vi "Vigia.vi"(7 "test module":T6, 10 "Robot":T1={"id"=0, "function"=enum."Attacker", "x"=0.0, "y"=0.0, "orientation"=0.0, "v_tangent"=0.0, "v_normal"=0.0, "v_ang"=0.0, "kick_x"=0.0, "kick_z"=0.0, "dribble"=FALSE, "Timestamp"=timestamp(0 s since 1904-01-01), "estimatives"={"est_v_tangent"=0.0, "est_v_normal"=0.0, "est_vx"=0.0, "est_vy"=0.0, "Pos Robot Est"=[]}, "dest_x_kick"=0.0, "dest_y_kick"=0.0, "Gap Coord"=[], "States"=enum."GoToTangent", "Path "=[], "Path  Smooth"=[], "Dest"=[], "Missões "=enum."Monitorar Comboio", "Agentes Disponíveis"=0.0, "Number"=0.0} {"Agentes Disponíveis" format="%#_13g"}, 11 "Al Input":T8={"our_robots"=[], "enemy_robots"=[], "balls"=[], "geometry"={"line_width"=0, "field_length"=0, "field_width"=0, "boundary_width"=0, "referee_width"=0, "goal_width"=0, "goal_depth"=0, "goal_wall_width"=0, "center_circle_radius"=0, "defense_radius"=0, "defense_stretch"=0, "free_kick_from_defense_dist"=0, "penalty_spot_from_field_line_dist"=0, "penalty_line_from_spot_dist"=0}, "IA Judge"={"stage"="", "command"="", "our_goalie_id"=0.0, "enemy_goalie_id"=0.0, "command enum"=enum."Halt", "Time"=enum."Azul"}, "Received Timestamp"=timestamp(0 s since 1904-01-01), "Events"={"Touch"=FALSE, "Ball out"=FALSE, "id touch"=0.0, "Ball out of \nVision"=FALSE, "Ball inside \nGoalie area"=FALSE, "Robot not responding"=FALSE, "Robots responding status"=[1.0, 1.0, 1.0, 1.0, 1.0, 1.0], "Enemy Ball \nPossession"=FALSE, "Pass State"=FALSE, "id end of pass"=0.0, "Kick"=FALSE, "Id ini Possession"=0.0, "Ball Possesion"=FALSE, "Id Possesion"=0.0, "Direct Kick"=FALSE, "2nd Strk Ativo"=FALSE}} {"enemy_robots"."Agentes Disponíveis" format="%#_13g"; "our_robots"."Agentes Disponíveis" format="%#_13g"}) -> (3 "Output Robot":T1={"id"=0, "function"=enum."Attacker", "x"=0.0, "y"=0.0, "orientation"=0.0, "v_tangent"=0.0, "v_normal"=0.0, "v_ang"=0.0, "kick_x"=0.0, "kick_z"=0.0, "dribble"=FALSE, "Timestamp"=timestamp(0 s since 1904-01-01), "estimatives"={"est_v_tangent"=0.0, "est_v_normal"=0.0, "est_vx"=0.0, "est_vy"=0.0, "Pos Robot Est"=[]}, "dest_x_kick"=0.0, "dest_y_kick"=0.0, "Gap Coord"=[], "States"=enum."GoToTangent", "Path "=[], "Path  Smooth"=[], "Dest"=[], "Missões "=enum."Monitorar Comboio", "Agentes Disponíveis"=0.0, "Number"=0.0} {"Agentes Disponíveis" format="%#_13g"})   [LabVIEW 2018]
uses:
  Core/AI Robot.ctl
  Functions Enum.ctl
  AttackerStates.ctl
  Path Planning/RRT/PathDests.ctl
  Path Planning/RRT/PathDest.ctl
  Core/AI Input.ctl
  Core/AI Ball.ctl
  Core/Field Size.ctl
  Core/AI Judge.ctl
  Command Enum.ctl
  Util/Events/Events.ctl
  Test/TestModule.ctl
  Util/Select None or Robot.ctl
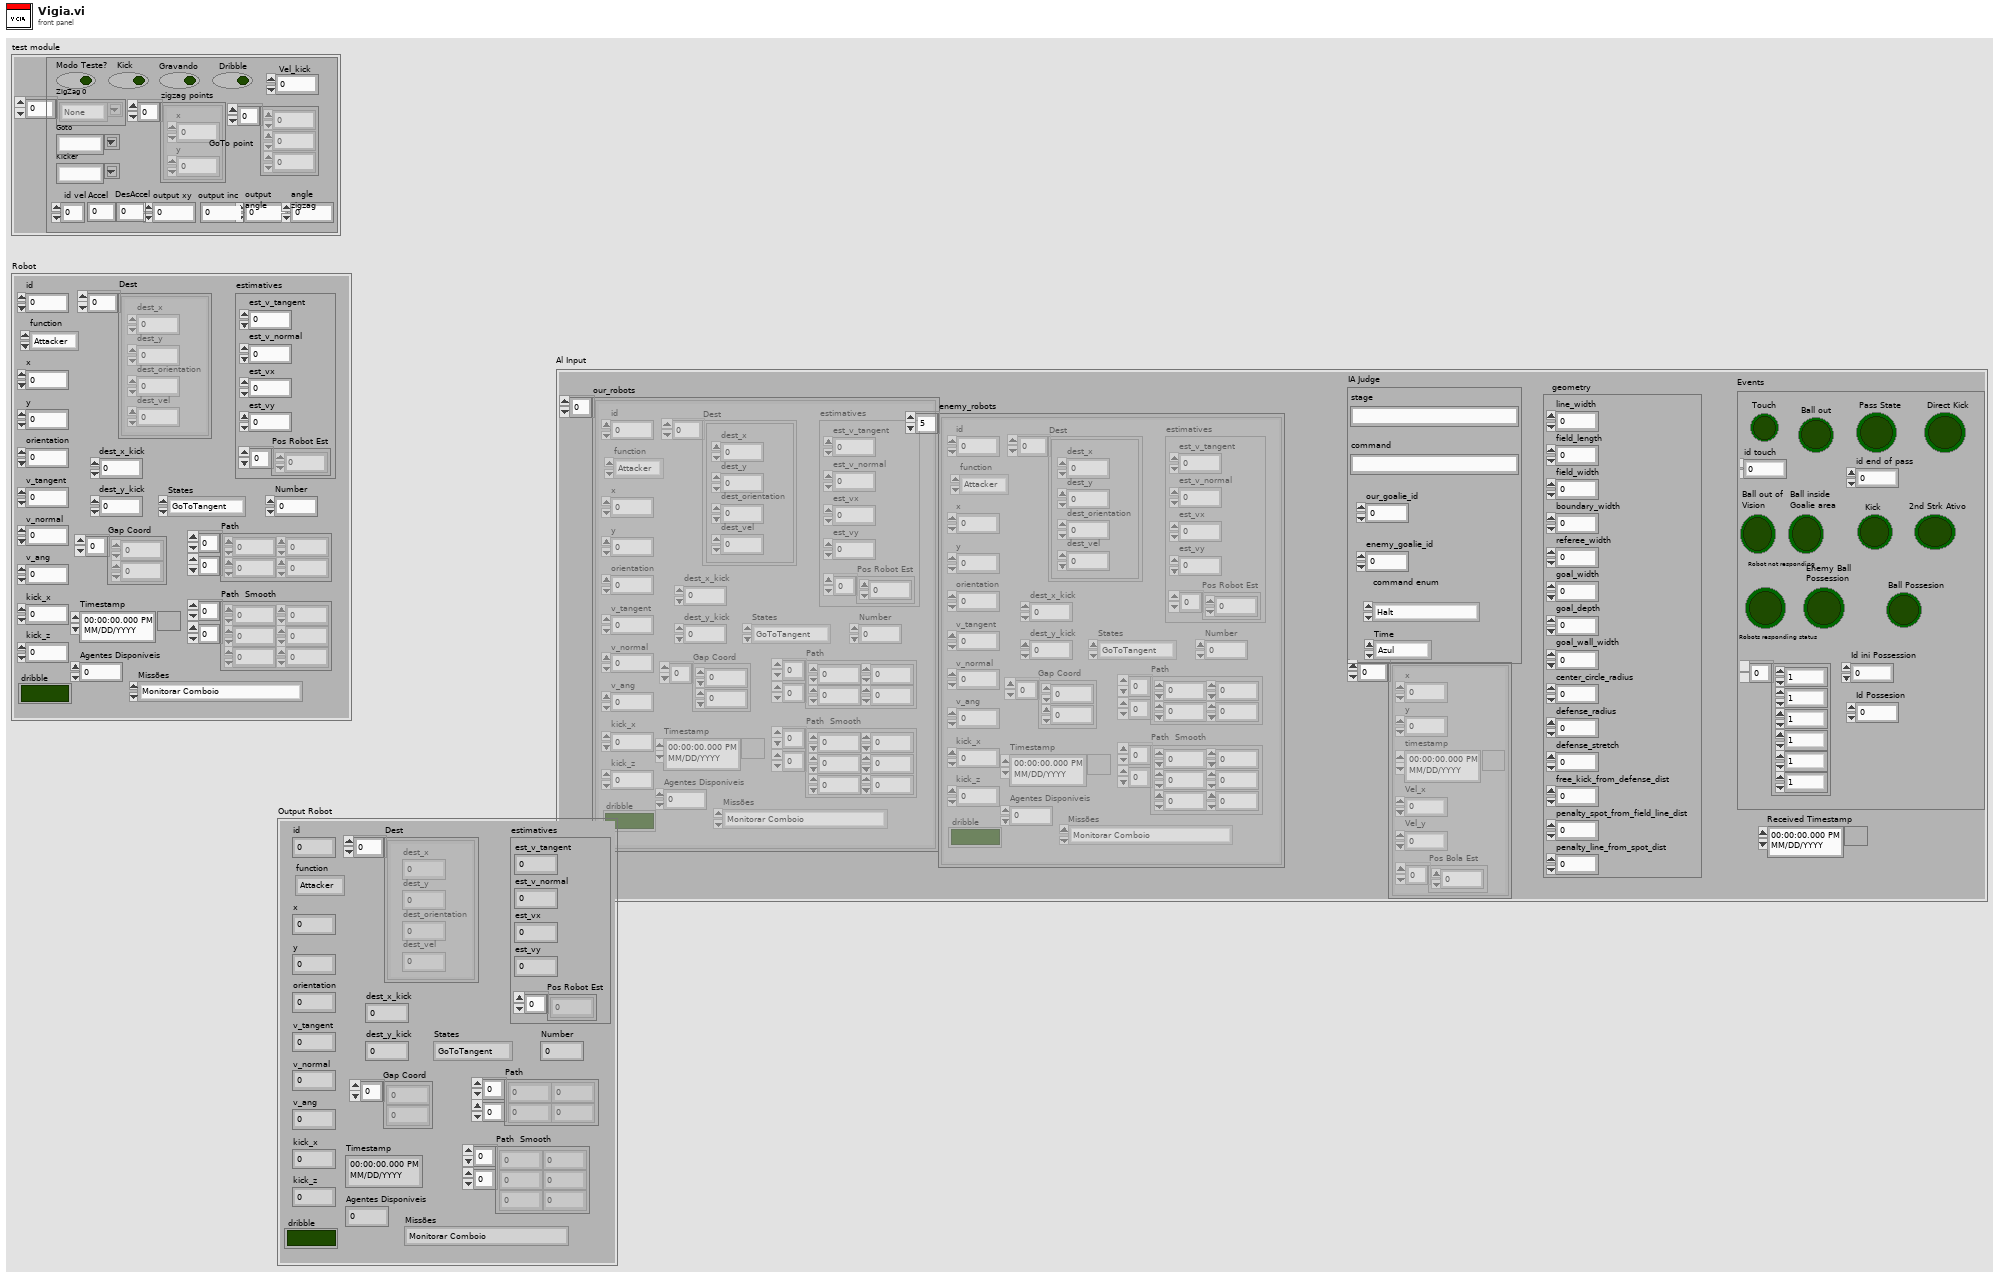
[diagram p1: front panel]
types:
  T1 = typedef "AI Robot.ctl" = cluster{"id":u32, "function":T2, "x":dbl, "y":dbl, "orientation":dbl, "v_tangent":dbl, "v_normal":dbl, "v_ang":dbl, "kick_x":dbl, "kick_z":dbl, "dribble":bool, "Timestamp":timestamp, "estimatives":cluster{"est_v_tangent":dbl, "est_v_normal":dbl, "est_vx":dbl, "est_vy":dbl, "Pos Robot Est":dbl[]}, "dest_x_kick":dbl, "dest_y_kick":dbl, "Gap Coord":dbl[], "States":T3, "Path ":dbl[][], "Path  Smooth":dbl[][], "Dest":T4, "Missões ":enum16{"Monitorar Comboio", "Realizar Segurança de Retaguarda", "Vigiar Área", "Reconhecimento de Área"}, "Agentes Disponíveis":dbl, "Number":dbl}
  T2 = typedef "Functions Enum.ctl" = enum16{"None", "Vigia", "2nd Striker", "Attacker", "Goalie", "Defender", "Striker", "Goto 0", "Dummy", "Kicker", "ZigZag 0", "ZigZag 1", "ZigZag 2", "ZigZag 3", "ZigZag 4", "ZigZag 5", "ZigZag 6", "ZigZag 7", "ZigZag 8", ""}
  T3 = typedef "AttackerStates.ctl" = enum16{"Pass", "GoToTangent", "BallGetting", "GoToKick", ""}
  T4 = typedef "PathDests.ctl" = T5[]
  T5 = typedef "PathDest.ctl" = cluster{"dest_x":dbl, "dest_y":dbl, "dest_orientation":dbl, "dest_vel":dbl}
  T6 = typedef "TestModule.ctl" = cluster{"Goto":T7, "ZigZag 0":T7[], "Kicker":T7, "Vel_kick":dbl, "Kick":bool, "Modo Teste?":bool, "GoTo point":dbl[], "zigzag points":cluster{"x":dbl, "y":dbl}[], " id vel":u32, "Dribble":bool, "Gravando":bool, "output xy":dbl, "output\nangle":dbl, "angle\nzigzag":dbl, "output inc":dbl, "Accel":dbl, "DesAccel":dbl}
  T7 = typedef "Select None or Robot.ctl" = string
  T8 = typedef "AI Input.ctl" = cluster{"our_robots":T1[], "enemy_robots":T1[], "balls":T9[], "geometry":T10, "IA Judge":T11, "Received Timestamp":timestamp, "Events":T13}
  T9 = typedef "AI Ball.ctl" = cluster{"x":dbl, "y":dbl, "timestamp":timestamp, "Vel_x":dbl, "Vel_y":dbl, "Pos Bola Est":dbl[]}
  T10 = typedef "Field Size.ctl" = cluster{"line_width":u32, "field_length":u32, "field_width":u32, "boundary_width":u32, "referee_width":u32, "goal_width":u32, "goal_depth":u32, "goal_wall_width":u32, "center_circle_radius":u32, "defense_radius":u32, "defense_stretch":u32, "free_kick_from_defense_dist":u32, "penalty_spot_from_field_line_dist":u32, "penalty_line_from_spot_dist":u32}
  T11 = typedef "AI Judge.ctl" = cluster{"stage":string, "command":string, "our_goalie_id":dbl, "enemy_goalie_id":dbl, "command enum":T12, "Time":enum16{"Azul", "Amarelo"}}
  T12 = typedef "Command Enum.ctl" = enum16{"Halt", "Stop", "Force Start", "PKA Normal Start", "Prepare Kickoff Ally", "PKE Normal Start", "Prepare Kickoff Enemy", "Prepare Penalty Ally", "PPA Normal Start", "Prepare Penalty Enemy", "PPE Normal Start", "Direct Free Enemy", "Direct Free Ally", "Indirect Free Enemy", "Indirect Free Ally", "Timeout Enemy", "Timeout Ally", "Goal Enemy", "Goal Ally", "Ball Placement Enemy", "Ball Placement Ally", "Normal Half Time", "Extra Time Break", "Extra Half Time", "None", "Post Game"}
  T13 = typedef "Events.ctl" = cluster{"Touch":bool, "Ball out":bool, "id touch":dbl, "Ball out of \nVision":bool, "Ball inside \nGoalie area":bool, "Robot not responding":bool, "Robots responding status":dbl[], "Enemy Ball \nPossession":bool, "Pass State":bool, "id end of pass":dbl, "Kick":bool, "Id ini Possession":dbl, "Ball Possesion":bool, "Id Possesion":dbl, "Direct Kick":bool, "2nd Strk Ativo":bool}
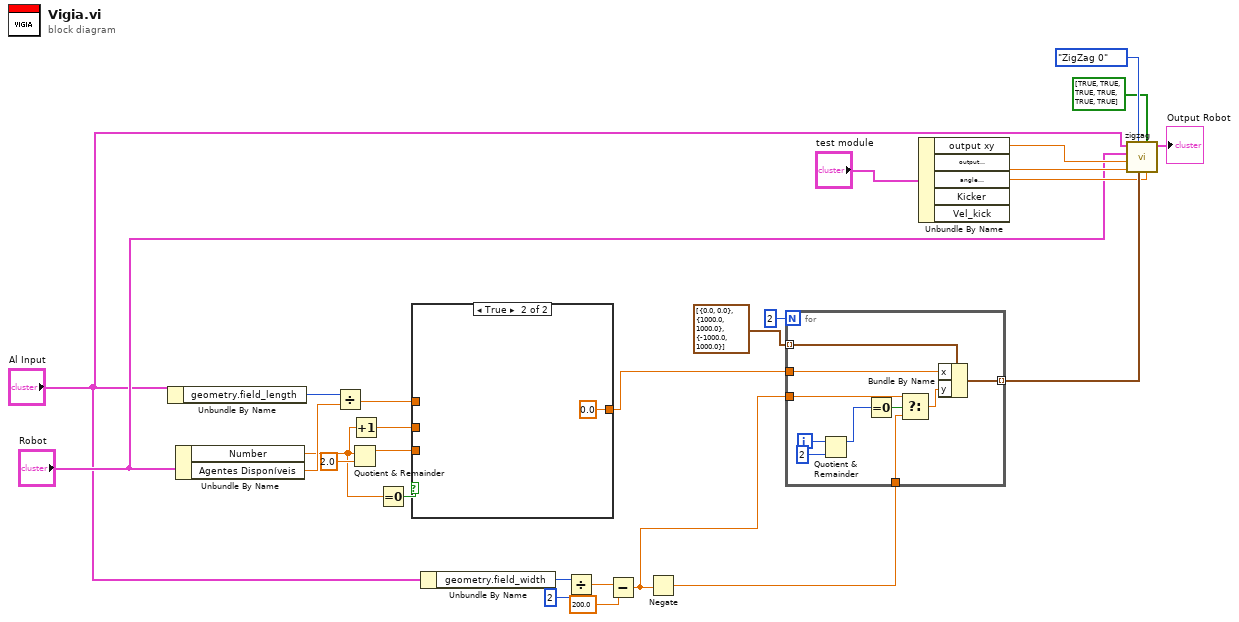
[diagram p0: block diagram]
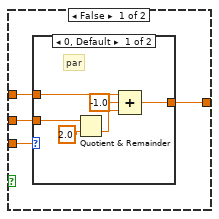
[diagram p2: hidden frame]
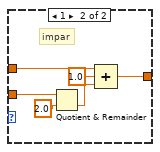
[diagram p3: hidden frame]
diagram:
  n1 = Unbundle By Name("Al Input") -> ("geometry.field_length"=w27:u32)
  n2 = Unbundle By Name("Robot") -> ("Number"=w20:dbl, "Agentes Disponíveis"=w26:dbl)
  n3 = Divide(x=w27, y=w26) -> (x/y=w22:dbl)
  n4 = Quotient & Remainder(x=w20, y=2.0) -> (x-y*floor(x/y)=w24:dbl)  [unwired: 1 out]
  n5 = Increment(x=w20) -> (x+1=w23:dbl)
  n6 = Equal To 0?(x=w20) -> (x = 0?=w21:bool)
  n7 = case shown="True" w21 {
    tunnel: w24 -> [w31 _]
    tunnel: w23 -> [w30 _]
    tunnel: w22 -> [w29 _]
    tunnel: [w28 0.0] -> w12
    frame False {
      n8 = case shown="0, Default" w31 {
        tunnel: w30 -> [w37 w43]
        tunnel: w29 -> [w34 w40]
        tunnel: [w32 w38] -> w28
        frame 0, Default {
          # "par"
          n9 = Quotient & Remainder(x=w37, y=2.0) -> (floor(x/y)=w35:dbl)  [unwired: 1 out]
          n10 = Compound Arithmetic op=ADD(w34, -1.0 ("value"), w35) -> (w32:dbl)
        }
        frame 1 {
          # "impar"
          n11 = Quotient & Remainder(x=w43, y=2.0) -> (floor(x/y)=w41:dbl)  [unwired: 1 out]
          n12 = Compound Arithmetic op=ADD(w40, 1.0 ("value"), w41) -> (w38:dbl)
        }
      }
    }
    frame True {
    }
  }
  n13 = Unbundle By Name("Al Input") -> ("geometry.field_width"=w19:u32)
  n14 = Divide(x=w19, y=u32 2) -> (x/y=w17:dbl)
  n15 = Subtract(x=w17, y=200.0) -> (x-y=w13:dbl)
  n16 = Negate(x=w13) -> (-x=w14:dbl)
  n17 = for {
    N: 2 -> [_]
    tunnel: cluster{"x":dbl, "y":dbl}[] [{"x"=0.0, "y"=0.0}, {"x"=1000.0, "y"=1000.0}, {"x"=-1000.0, "y"=1000.0}] ("points 3") -> [w54] mode=indexing
    tunnel: w14 -> [w49]
    tunnel: w13 -> [w48]
    tunnel: w12 -> [w47]
    tunnel: [w45] -> w10 mode=indexing
    i -> [w53]
    n18 = Quotient & Remainder(x=w53, y=2) -> (x-y*floor(x/y)=w50:i32)  [unwired: 1 out]
    n19 = Equal To 0?(x=w50) -> (x = 0?=w51:bool)
    n20 = Select(t=w48, s=w51, f=w49) -> (s? t:f=w46:dbl)
    n21 = Bundle By Name(cluster=w54, "x"=w47, "y"=w46) -> (w45:cluster{"x":dbl, "y":dbl})
  }
  n22 = Unbundle By Name("test module") -> ("output xy"=w7:dbl, "output\nangle"=w8:dbl, "angle\nzigzag"=w6:dbl)  [unwired: 2 out]
  n23 = call "zigzag.vi"("angulo"=w6, "Change point by ID"=bool[] [TRUE, TRUE, TRUE, TRUE, TRUE, TRUE], "points 3"=w10, "ZigZag Number"=Functions_Enum."ZigZag 0" ("y"), "output angle"=w8, "output xy"=w7, "Current Robot"="Robot", "Al Input"="Al Input") -> ("Output Robot"=→"Output Robot":T1)  [unwired: 1 in, 2 out]
